vi "带延迟的反馈节点.vi"() -> ()   [LabVIEW 2020]
panel:
  out "数值":dbl
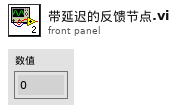
[diagram p1: front panel]
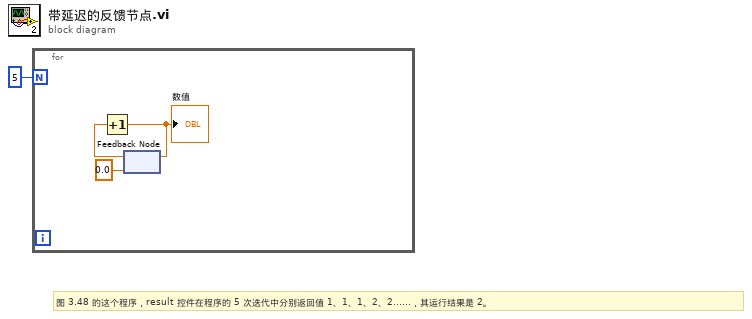
[diagram p0: block diagram]
diagram:
  # "图 3.48 的这个程序，result 控件在程序的 5 次迭代中分别返回值 1、1、1、2、2......，其运行结果是 2。"
  n1 = for {
    N: 5 -> [_]
    n2 = feedback #1 ("反馈节点")(0.0) -> (w4:dbl)
    n3 = Increment(x=w4) -> (x+1=w2:dbl)
    "数值" <- w2
    n4 = feedback-in #1(w2) -> ()
  }
